vi "Create User Event - Stop.vi"(8 "error in (no error)":T1 caption="entrée d'erreur (pas d'erreur)") -> (0 "error out":T1 caption="sortie d'erreur", 3 "Événement utilisateur - Arrêter":refnum<user-event>)   [LabVIEW 2018, in "User Event - Stop.lvlib"]
doc: "Créer un événement utilisateur booléen qui sera utilisé pour arrêter la boucle d'événement à partir de la boucle de gestion de messages."
uses:
  User Event - Stop.lvlib
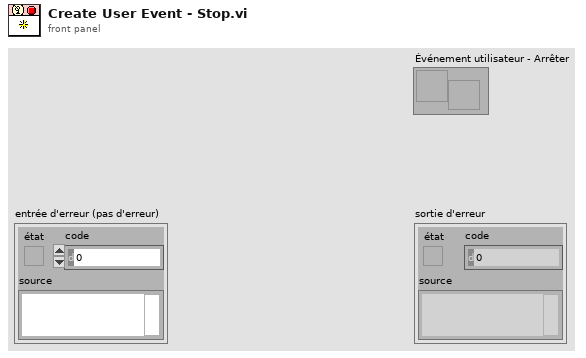
[diagram p1: front panel]
types:
  T1 = cluster{"état":bool, "code":i32, "source":string}
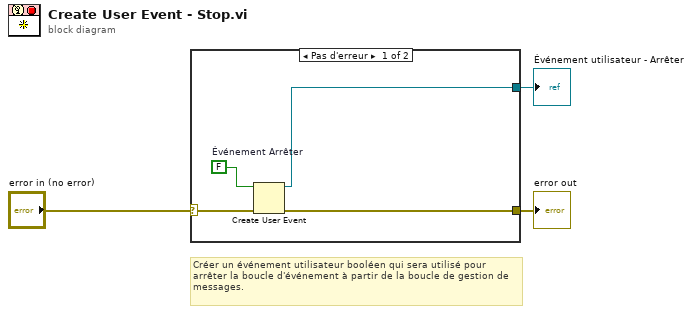
[diagram p0: block diagram]
diagram:
  # "Créer un événement utilisateur booléen qui sera utilisé pour arrêter la boucle d'événement à partir de la boucle de gestion de messages."
  n1 = case shown="Pas d'erreur" "error in (no error)" {
    selector: "error in (no error)" -> [w4 w8]
    tunnel: [w7 _] -> w3
    tunnel: [w5 w8] -> w2
    frame No Error {
      w6 = FALSE  # Événement Arrêter
      n2 = Create User Event(user event datatype=w6, error in=w4) -> (user event=w7:refnum<user-event>, error out=w5:errorcluster)
    }
    frame Error {
    }
  }
  "Événement utilisateur - Arrêter" <- w3
  "error out" <- w2
